vi "Init.vi"(0 "Arduino Resource in":T1, 11 "error in (no error)":errorcluster) -> (4 "Arduino Resource Out":T1, 15 "error out":errorcluster)   [LabVIEW 2012, in "Digital Compass HMC5883L.lvlib"]
doc: "Sets the mode to Continuous- Measurement Mode."
uses:
  Digital Compass HMC5883L.lvlib
  <vilib>/LabVIEW Interface for Arduino/Type Defs/Arduino Resource.ctl
  <vilib>/LabVIEW Interface for Arduino/Type Defs/Board Type.ctl
  Registers.ctl
  <vilib>/LabVIEW Interface for Arduino/LabVIEW Interface for Arduino.lvlib
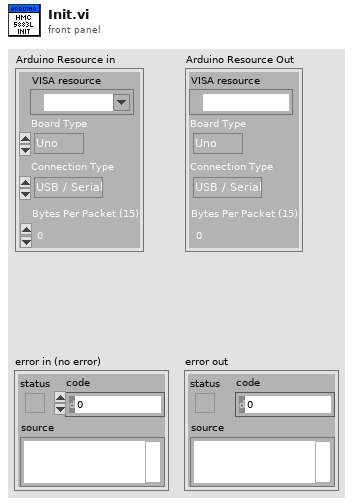
[diagram p1: front panel]
types:
  T1 = typedef "LabVIEW Interface for Arduino.lvlib/Arduino Resource.ctl" = cluster{"VISA resource":refnum<visa-resource-name>, "Board Type":T2, "Connection Type":enum8{"USB / Serial"}, "Bytes Per Packet (15)":u8}
  T2 = typedef "LabVIEW Interface for Arduino.lvlib/Board Type.ctl" = enum16{"Uno", "Dimuelanove w/Atmega 328", "Mega 2560"}
  T3 = typedef "Digital Compass HMC5883L.lvlib/Registers.ctl" = enum16{"Config A", "Config B", "Mode", "X MSB", "X LSB", "Z MSB", "Z LSB", "Y MSB", "Y LSB", "Status", "ID A", "ID B", "ID C"}
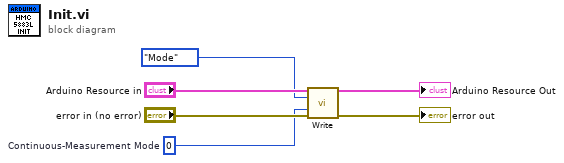
[diagram p0: block diagram]
diagram:
  w4 = u8 0  # Continuous-Measurement Mode
  n1 = call "Write.vi"("Arduino Resource in"="Arduino Resource in", "Register"=Registers."Mode", "Value"=w4, "error in (no error)"="error in (no error)") -> ("Arduino Resource Out"=→"Arduino Resource Out":T1, "error out"=→"error out":errorcluster)  [unwired: 10 in]
